vi "trial1_fromSpotSizeProgram1.vi"() -> ()   [LabVIEW 2017]
panel:
  in  "Step Size [um]":i32=10
  in  "Axis":i32=1
  in  "Rep Rate [Hz]":dbl=500.0
  out "Shots":dbl
  in  "Averaging Time [s]":dbl=0.1
  out "Current Point":i32
  out "Slide":i32(slide) scale=0.0..100.0
  out "Current Position [mm]":dbl
  in  "Axis initial position [mm]":dbl
  out "Axis final Position [mm]":dbl
  in  "Data Points (100 default)":i32=100
  in  "Collect Data!":bool
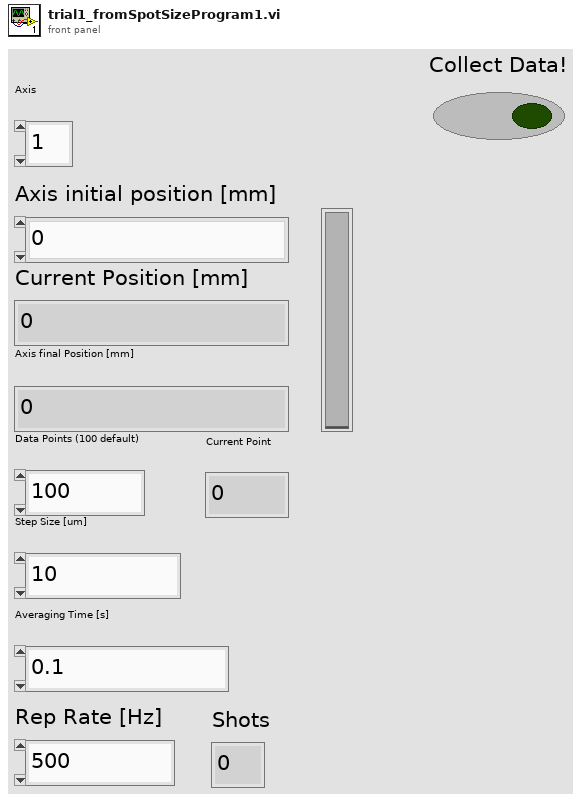
[diagram p1: front panel]
types:
  T1 = cluster{"input XON/XOFF":bool, "input HW Handshake":bool, "input alt HW HShk":bool, "output XON/XOFF":bool, "output HW Handshake":bool, "output alt HW HShk":bool, "XOFF byte":u8, "XON byte":u8, "parity error byte":u16}
  T2 = enum16{"no parity", "odd parity", "even parity", "mark parity", "space parity"}
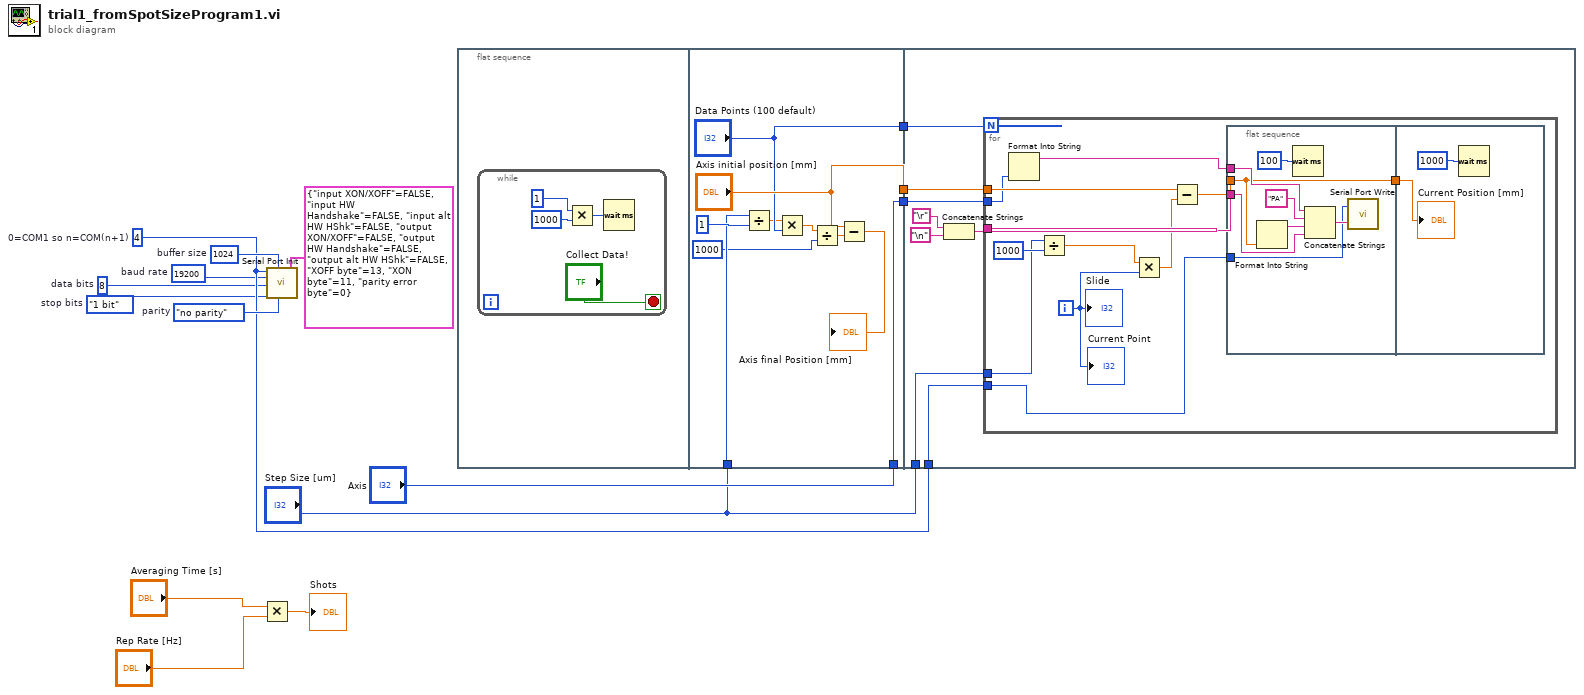
[diagram p0: block diagram]
diagram:
  w3 = u32 19200  # baud rate
  w2 = u16 8  # data bits
  w1 = enum16{"1 bit", "1.5 bits", "2 bits"}."1 bit"  # stop bits
  w7 = T2."no parity"  # parity
  w5 = 4  # 0=COM1 so n=COM(n+1)
  w6 = u16 1024  # buffer size
  n1 = Multiply(x="Averaging Time [s]", y="Rep Rate [Hz]") -> (x*y=→"Shots":dbl)
  n2 = call <vilib>:"Serial Port Init.vi"("flow control etc."=T1 {"input XON/XOFF"=FALSE, "input HW Handshake"=FALSE, "input alt HW HShk"=FALSE, "output XON/XOFF"=FALSE, "output HW Handshake"=FALSE, "output alt HW HShk"=FALSE, "XOFF byte"=13, "XON byte"=11, "parity error byte"=0}, "parity"=w7, "buffer size"=w6, "stop bits"=w1, "data bits"=w2, "baud rate"=w3, "port number"=w5) -> ()  [unwired: 1 out]
  n3 = flat-sequence {
    tunnel: ["Data Points (100 default)"] -> w15
    tunnel: "Axis" -> [w29]
    tunnel: ["Axis initial position [mm]"] -> w14
    tunnel: "Step Size [um]" -> [w26]
    tunnel: [w29] -> w13
    tunnel: w15 -> [w37]
    tunnel: w14 -> [w36]
    tunnel: "Step Size [um]" -> [w35]
    tunnel: w13 -> [w34]
    tunnel: w5 -> [w30]
    frame #0 {
      n4 = while {
        stop <- "Collect Data!" stop-if-true
        n5 = Multiply(x=1, y=1000) -> (x*y=w19:i32)
        n6 = Wait (ms)(milliseconds to wait=w19) -> ()  [unwired: 1 out]
      }
    }
    frame #1 {
      n7 = Divide(x=w26, y=1) -> (x/y=w24:dbl)
      n8 = Multiply(x=w24, y="Data Points (100 default)") -> (x*y=w22:dbl)
      n9 = Divide(x=w22, y=1000) -> (x/y=w21:dbl)
      n10 = Subtract(x="Axis initial position [mm]", y=w21) -> (x-y=→"Axis final Position [mm]":dbl)
    }
    frame #2 {
      n11 = Concatenate Strings("\r", "\n") -> (w31:string)
      n12 = for {
        N: w37 -> [_]
        tunnel: w36 -> [w48]
        tunnel: w35 -> [w44]
        tunnel: w34 -> [w40]
        tunnel: w31 -> [w41]
        tunnel: w30 -> [w38]
        i -> [w49]
        n13 = Format Into String(w40) -> (resulting string=w39:string)  [unwired: 3 in, 1 out]
        n14 = Divide(x=w44, y=1000) -> (x/y=w43:dbl)
        n15 = Multiply(x=w43, y=w49) -> (x*y=w47:dbl)
        n16 = Subtract(x=w48, y=w47) -> (x-y=w46:dbl)
        n17 = flat-sequence {
          tunnel: w46 -> [w52]
          tunnel: [w52] -> w42
          tunnel: w41 -> [w54]
          tunnel: w39 -> [w53]
          tunnel: w38 -> [w50]
          tunnel: w42 -> [w58]
          frame #0 {
            n18 = Format Into String(w52) -> (resulting string=w51:string)  [unwired: 3 in, 1 out]
            n19 = Wait (ms)(milliseconds to wait=u32 100) -> ()  [unwired: 1 out]
            n20 = Concatenate Strings(w53, "PA" ("Substring"), w51, w54) -> (w56:string)
            n21 = call <vilib>:"Serial Port Write.vi"("string to write"=w56, "port number"=w50) -> ()  [unwired: 1 out]
          }
          frame #1 {
            n22 = Wait (ms)(milliseconds to wait=u32 1000) -> ()  [unwired: 1 out]
            "Current Position [mm]" <- w58
          }
        }
        "Current Point" <- w49
        "Slide" <- w49
      }
    }
  }
